vi "Pipe Var Intf - Write Variable Data.vi"(4 "columns":i32, 5 "write block size (10k)":i32=10000, 6 "rows":i32, 7 "timeout [ms]":i32=3000, 8 "error in (no error)":errorcluster, 9 "data type":T1, 10 "data":u8[](array[numeric]), 11 "pipe handle":i32) -> (0 "error out":errorcluster, 3 "pipe handle out":i32)   [LabVIEW 2020, in "GOLPI library.lvlib"]
doc: "Tries to write variable binary data with header for the Pipe Variable Interface."
uses:
  GOLPI library.lvlib
  Pipe Var Intf - Data Type.ctl
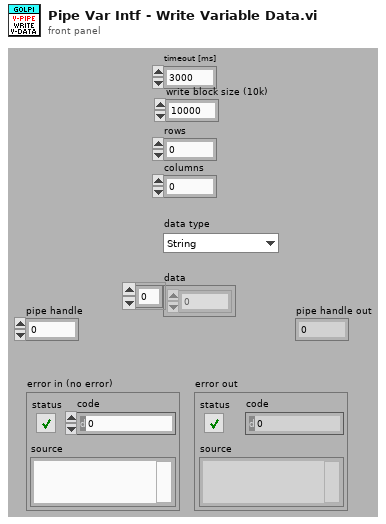
[diagram p1: front panel]
types:
  T1 = typedef "GOLPI library.lvlib/Pipe Var Intf - Data Type.ctl" = enum16{"String", "int32", "uint32", "double", "cplx double", "single", "cplx single"}
  T2 = enum16{"big-endian, network order", "native, host order", "little-endian"}
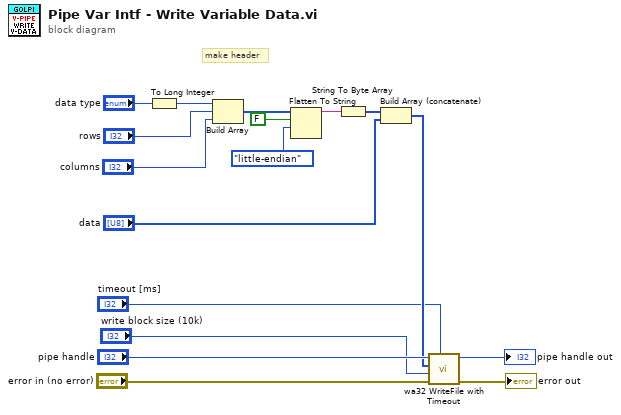
[diagram p0: block diagram]
diagram:
  # "make header"
  n1 = To Long Integer(number="data type") -> (32bit integer=w14:i32)
  n2 = Build Array(w14, "rows", "columns") -> (w10:i32[])
  n3 = Flatten To String(anything=w10, prepend array or string size? (T)=FALSE, byte order (0:big-endian, network order)=T2."little-endian") -> (data string=w7:string)  [unwired: 1 in, 2 out]
  n4 = String To Byte Array(string=w7) -> (unsigned byte array=w6:u8[])
  n5 = Build Array (concatenate)(w6, "data") -> (w4:u8[])
  n6 = call "wa32 WriteFile with Timeout.vi"("timeout [ms]"="timeout [ms]", "error in (no error)"="error in (no error)", "write block size (10k)"="write block size (10k)", "data"=w4, "pipe handle"="pipe handle") -> ("error out"=→"error out":errorcluster, "pipe handle out"=→"pipe handle out":i32)  [unwired: 4 in, 1 out]
